vi "Thingworx_Write_num.vi"(9 "Numeric":dbl, 11 "Thingworx":string(xcontrol)) -> ()   [LabVIEW 2020]
uses:
  TW_XControl.xctl
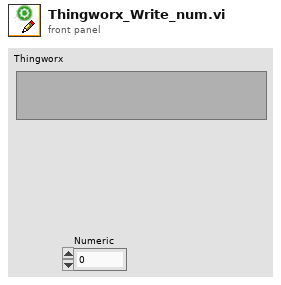
[diagram p1: front panel]
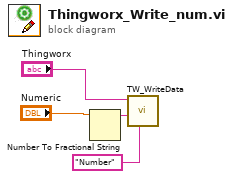
[diagram p0: block diagram]
diagram:
  n1 = Number To Fractional String(number="Numeric") -> (F-format string=w2:string)  [unwired: 3 in]
  n2 = call "TW_WriteData.vi"("Type"="Number", "value"=w2, "Property"="Thingworx") -> ()  [unwired: 9 in]
